vi "SaveMean_Example.vi"() -> ()   [LabVIEW 2019]
doc: "This example shows how to record an image sequence, get the mean of that sequence and save it to file afterwards.\nIt is a good starting point for writing own applications.\nBut it will not be fail save, i.e. doesnt react on errors, just handles them forward to the end\n\nUsage:\nSelect your required image count you want to average over before you start the program.\nOnce started, the camera class will be initialized and images will be recorded automatically.\nTWhen acquisition has finished the mean image is read and shown.\nNow you can crop the image using the ROI parameters and select a file path.\nBy clicking save, the mean image is saved with the selected file format using the current roi setting\nThis also finishes the program and will force an exit of the camera class"
uses:
  camera/Camera.lvclass
  pco.recorder/Recorder.lvlib
  <vilib>/picture/picture.llb/Draw 8-Bit Pixmap.vi
  <vilib>/picture/picture.llb/Draw True-Color Pixmap.vi
panel:
  out "colormap(U8)":u32[](array[numeric])
  out "Image(U16)":u16[][](graph)
  in  "Zoom [%]":i32(slide)=26 min=10 max=200 step=5 scale=10.0..200.0
  out "Image":picture
  out "rawImage":u16[][](array[numeric])
  in  "data_format":T1(ring)=enum."Mono16"
  in  "Image Index":u32 max=99
  in  "saveImages":bool
  in  "SavePath":path
  out "Recorded Images":u32
  in  "Quit":bool
  in  "cropY1":u64=2 min=2 max=2048 step=1
  in  "cropX1":u64=2 min=2 max=2048 step=1
  in  "cropY0":u64=1 min=1 max=2047 step=1
  in  "cropX0":u64=1 min=1 max=2047 step=1
  out "Image Height":u16
  out "Image Width":u16
  in  "dwImgCount":u32=10 caption="Required Number of Images" max=4023
  out "Error":errorcluster {"code" format="%x"}
  # "This example shows how to record an image sequence, get the mean of that sequence and save it to file afterwards.\nIt is a good starting point for writing own applications.\nBut it will not be fail save, i.e. doesnt react on errors, just handles them forward to the end\n\nUsage:\nSelect your required image count you want to average over before you start the program.\nOnce started, the camera class will be initialized and images will be recorded automatically.\nTWhen acquisition has finished the mean image is read and shown.\nNow you can crop the image using the crop parameters and select a file path.\nBy clicking save, the mean image is saved with the selected file format using the current roi setting\nThis also finishes the program and will force an exit of the camera class"
  # "pco.labview"
  # "Camera Setup"
  # "Recording Control"
  # "Parameters for image readout"
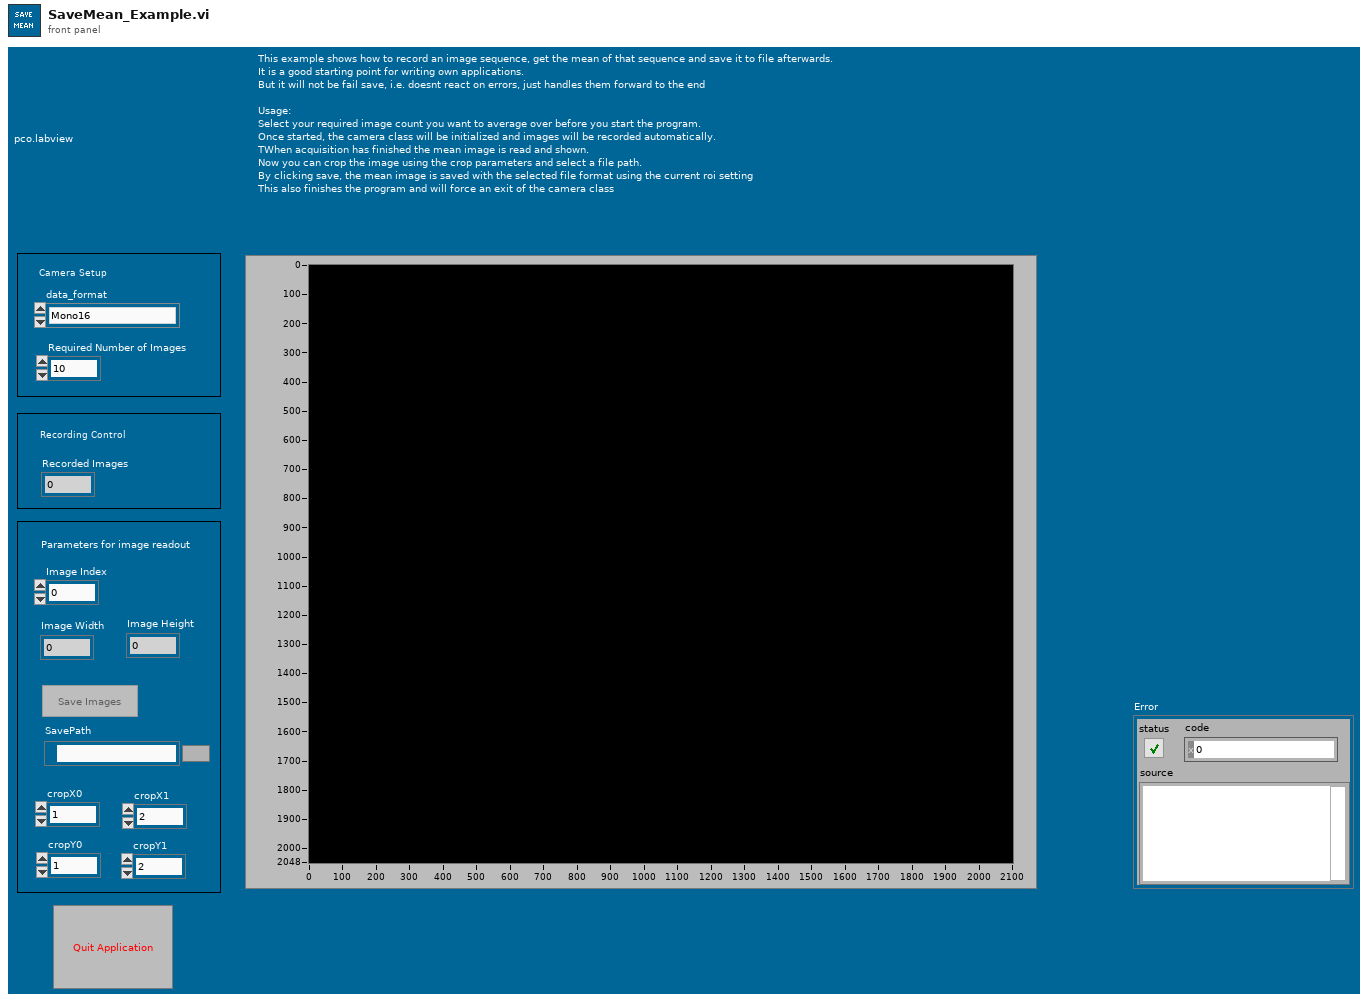
[diagram p1: front panel]
types:
  T1 = enum16{"Undefined", "Mono8", "Mono16", "BGRA8", "RGBA8", "BGRA16", "RGBA16", "CompressedMono8"}
  T2 = enum8{"Enabled", "Disabled", "Disabled and Grayed Out"}
  T3 = enum16{"sequence", "sequence non blocking", "ring buffer", "fifo", "tif", "multitif", "pcoraw", "b16", "dicom", "multidicom", "camram_ring", "camram_segment"}
  T4 = cluster{"wVersion":u16, "dwIMAGE_COUNTER":u32, "dwIMAGE_TIME_US":u32, "lvTimestamp":timestamp, "bIMAGE_TIME_STATUS":u8, "wEXPOSURE_TIME_BASE":u16, "dwEXPOSURE_TIME":u32, "dwFRAMERATE_MILLIHZ":u32, "sSENSOR_TEMPERATURE":i16, "wIMAGE_SIZE_X":u16, "wIMAGE_SIZE_Y":u16, "bBINNING_X":u8, "bBINNING_Y":u8, "dwSENSOR_READOUT_FREQUENCY":u32, "wSENSOR_CONV_FACTOR":u16, "dwCAMERA_SERIAL_NO":u32, "wCAMERA_TYPE":u16, "bBIT_RESOLUTION":u8, "bSYNC_STATUS":u8, "wDARK_OFFSET":u16, "bTRIGGER_MODE":u8, "bDOUBLE_IMAGE_MODE":u8, "bCAMERA_SYNC_MODE":u8, "bIMAGE_TYPE":u8, "wCOLOR_PATTERN":u16, "wCAMERA_SUBTYPE":u16, "dwEVENT_NUMBER":u32, "wIMAGE_SIZE_X_Offset":u16, "wIMAGE_SIZE_Y_Offset":u16, "bREADOUT_MODE":u8}
  T5 = typedef "Camera.lvclass/binning.ctl" = cluster{"vert":u16, "horz":u16, "mode":u16}
  T6 = cluster{"exposure_time_s":dbl, "delay_time_s":dbl, "roi":cluster{"x0":u64, "y0":u64, "x1":u64, "y1":u64}, "timestamp_mode":u16, "pixelrate":u32, "conversion_factor":sgl, "trigger_mode":u16, "acquire_mode":u16, "acquire_sequence_number":u32, "metadata_mode":u16, "noisefilter_mode":u16, "pixel_format":u32, "binning":T5, "auto_exposure":cluster{"region":u16, "min_exposure_s":dbl, "max_exposure_s":dbl}}
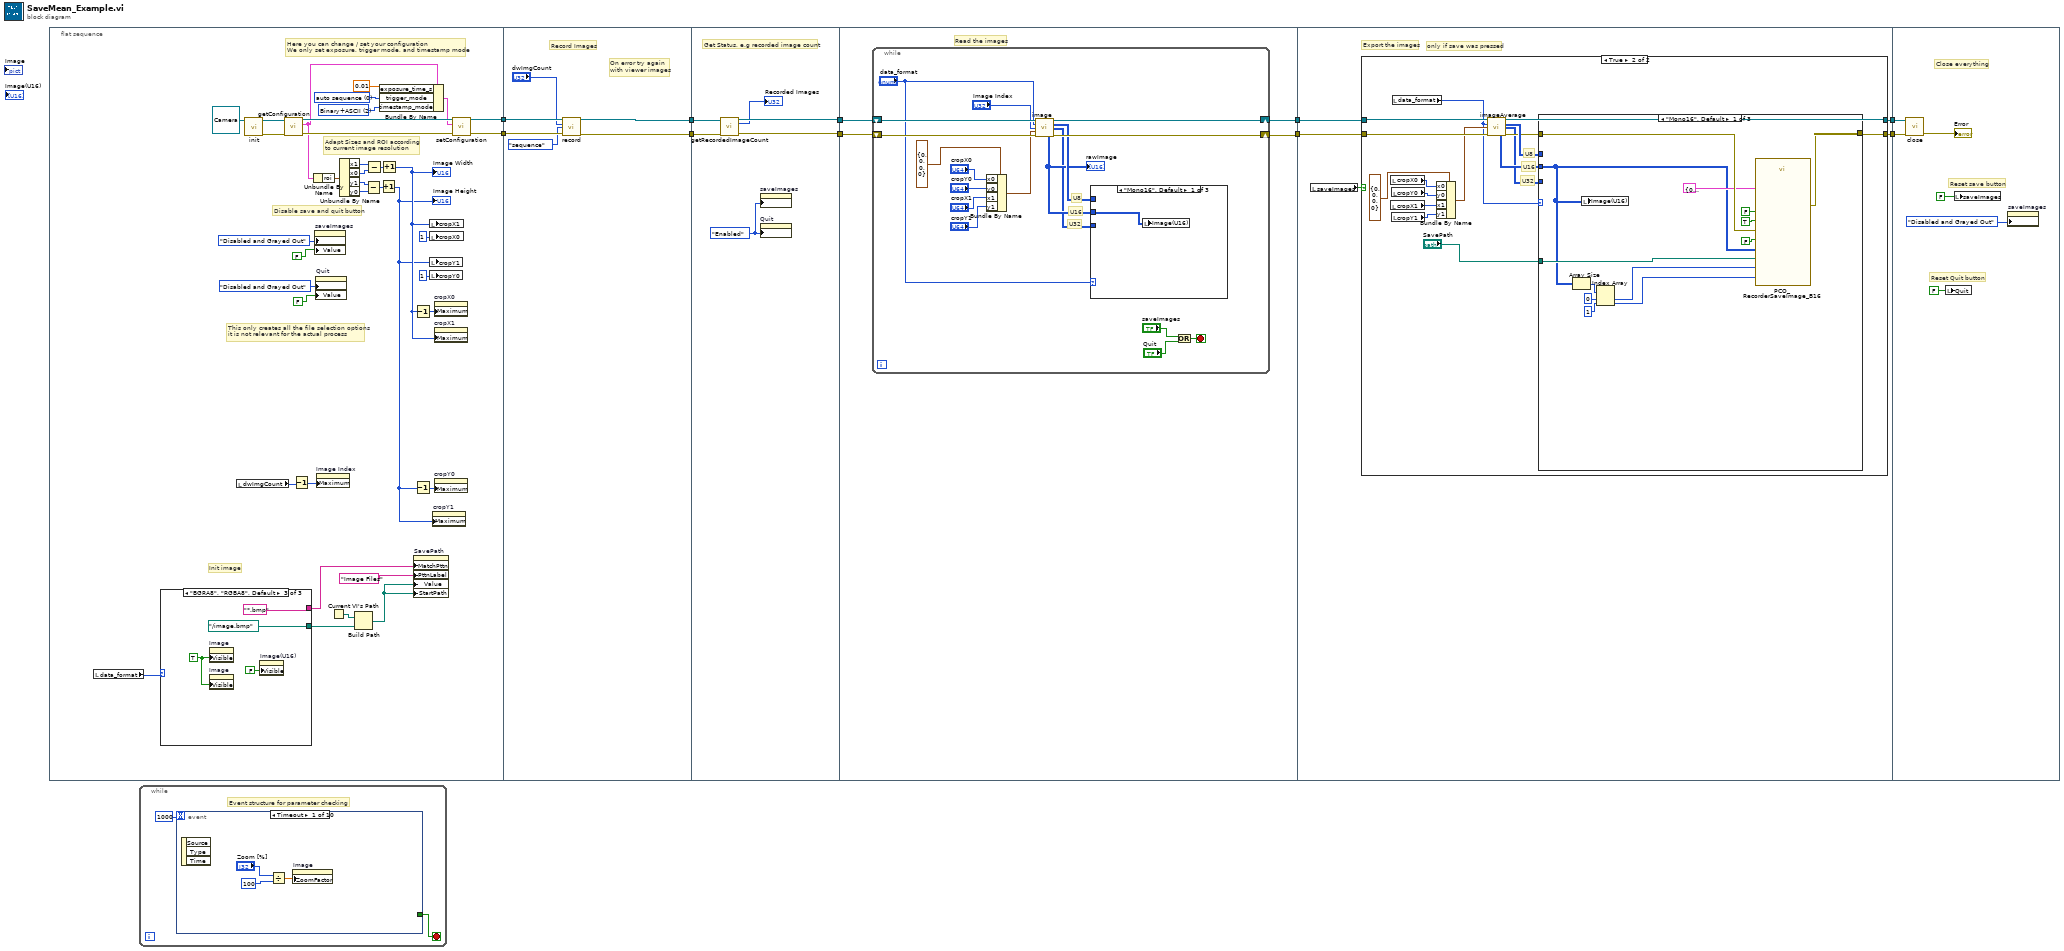
[diagram p0: block diagram]
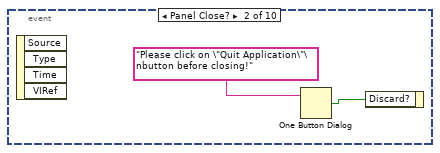
[diagram p2: hidden frame]
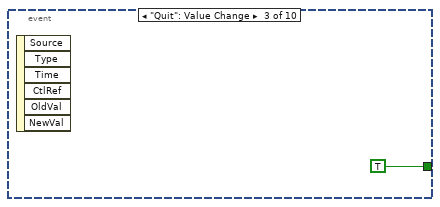
[diagram p3: hidden frame]
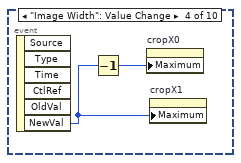
[diagram p4: hidden frame]
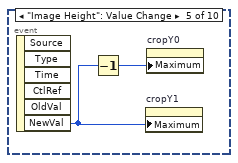
[diagram p5: hidden frame]
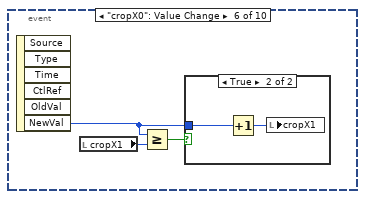
[diagram p6: hidden frame]
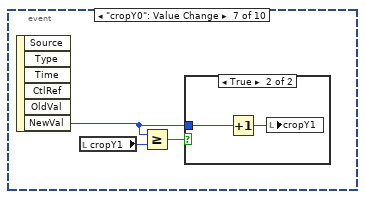
[diagram p8: hidden frame]
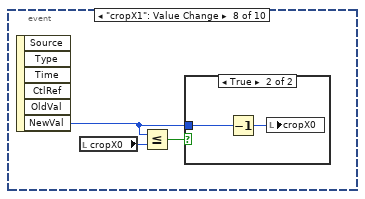
[diagram p10: hidden frame]
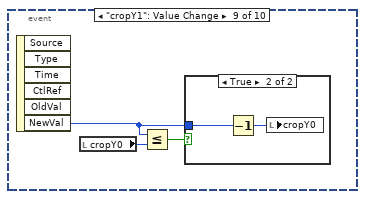
[diagram p12: hidden frame]
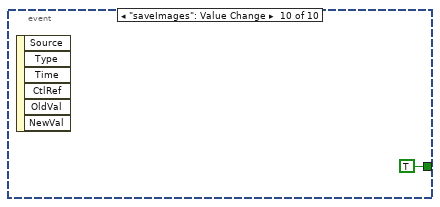
[diagram p14: hidden frame]
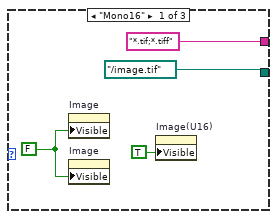
[diagram p15: hidden frame]
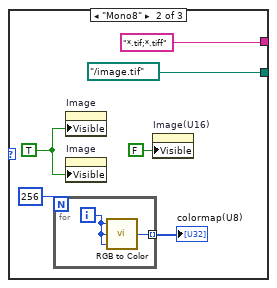
[diagram p16: hidden frame]
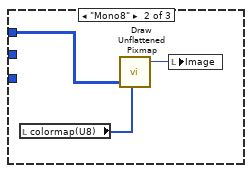
[diagram p17: hidden frame]
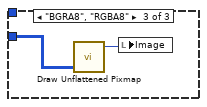
[diagram p18: hidden frame]
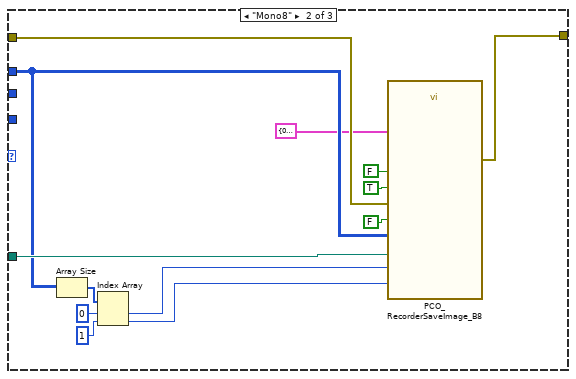
[diagram p20: hidden frame]
diagram:
  n1 = flat-sequence {
    tunnel: [w38] -> w10
    tunnel: [w37] -> w9
    tunnel: w10 -> [w69]
    tunnel: w9 -> [w68]
    tunnel: [w66] -> w8
    tunnel: [w65] -> w7
    tunnel: w8 -> [w75]
    tunnel: w7 -> [w74]
    tunnel: [w73] -> w6
    tunnel: [w72] -> w5
    tunnel: w6 -> [w78]
    tunnel: w5 -> [w79]
    tunnel: [w77] -> w4
    tunnel: [w76] -> w2
    tunnel: w4 -> [w107]
    tunnel: [w106] -> w3
    tunnel: w2 -> [w105]
    tunnel: [w104] -> w1
    tunnel: w3 -> [w180]
    tunnel: w1 -> [w179]
    frame #0 {
      w22 = u16 2 items=["OFF", "Binary", "Binary+ASCII", "ASCII"] ("TimestampMode")
      w44 = u16 0 items=["auto sequence"=0, "software trigger"=1, "external exposure start & software trigger"=2, "external exposure control"=3, "external synchronized"=4, "fast external exposure control"=5, "external CDS control"=6, "slow external exposure control"=7, "external synchronized HDSDI"=258] ("TriggerMode")
      # "Here you can change / set your configuration\nWe only set exposure, trigger mode, and timestamp mode"
      # "Init image"
      # "This only creates all the file selection options\nit is not relevant for the actual process"
      # "Adapt Sizes and ROI according\nto current image resolution"
      # "Disable save and quit button"
      n2 = local read "data_format"() -> (w14:T1)
      n3 = case shown="\"BGRA8\", \"RGBA8\", Default" w14 {
        tunnel: [path "../image.tif" ("SavePath") path "../image.tif" ("SavePath") path "../image.bmp" ("SavePath")] -> w13
        tunnel: ["*.tif;*.tiff" ("pattern (all files)") "*.tif;*.tiff" ("pattern (all files)") "*.bmp" ("pattern (all files)")] -> w12
        frame "Mono16" {
          w50 = FALSE ("Visible")
          n4 = property on="Image" class="Pict"("Visible"=w50) -> ()  [unwired: 2 in, 2 out]
          n5 = property on="Image" class="Pict"("Visible"=w50) -> ()  [unwired: 2 in, 2 out]
          n6 = property on="Image(U16)" class="IntGraph (strict)"("Visible"=TRUE) -> ()  [unwired: 2 in, 2 out]
        }
        frame "Mono8" {
          w56 = TRUE ("Visible")
          n7 = for {
            N: 256 -> [_]
            tunnel: [w58] -> w55 mode=indexing
            i -> [w59]
            n8 = call <vilib>:"RGB to Color.vi"("B"=w59, "G"=w59, "R"=w59) -> ("Color"=w58:u32)
          }
          "colormap(U8)" <- w55
          n9 = property on="Image" class="Pict"("Visible"=w56) -> ()  [unwired: 2 in, 2 out]
          n10 = property on="Image" class="Pict"("Visible"=w56) -> ()  [unwired: 2 in, 2 out]
          n11 = property on="Image(U16)" class="IntGraph (strict)"("Visible"=FALSE) -> ()  [unwired: 2 in, 2 out]
        }
        frame "BGRA8", "RGBA8", Default {
          w63 = TRUE ("Visible")
          n12 = property on="Image" class="Pict"("Visible"=w63) -> ()  [unwired: 2 in, 2 out]
          n13 = property on="Image" class="Pict"("Visible"=w63) -> ()  [unwired: 2 in, 2 out]
          n14 = property on="Image(U16)" class="IntGraph (strict)"("Visible"=FALSE) -> ()  [unwired: 2 in, 2 out]
        }
      }
      n15 = local read "dwImgCount"() -> (w15:u32)
      n16 = call-dynamic "init.vi"("Camera in"=refnum<class "Camera.lvclass"> refnum ("PCOCamera in")) -> ("Camera out"=w46:refnum<class "Camera.lvclass">, "error out"=w45:errorcluster)  [unwired: 8 in]
      n17 = call-dynamic "getConfiguration.vi"("error in (no error)"=w45, "Camera in"=w46) -> ("error out"=w42:errorcluster, "configuration"=w32:T6, "Camera out"=w43:refnum<class "Camera.lvclass">)  [unwired: 7 in]
      n18 = Decrement(x=w15) -> (x-1=w16:u32)
      n19 = Unbundle By Name(w32) -> ("roi"=w31:cluster{"x0":u64, "y0":u64, "x1":u64, "y1":u64})
      n20 = property on="saveImages" class="Bool (strict)"("DisabledEnum"=T2."Disabled and Grayed Out" ("Disabled"), "Value"=FALSE ("Stop")) -> ()  [unwired: 2 in, 2 out]
      n21 = property on="Quit" class="Bool (strict)"("DisabledEnum"=T2."Disabled and Grayed Out" ("Disabled"), "Value"=FALSE ("Stop")) -> ()  [unwired: 2 in, 2 out]
      n22 = property on="Image Index" class="DigNum (strict)"("Maximum"=w16) -> ()  [unwired: 2 in, 2 out]
      n23 = Current VI's Path() -> (path=w19:path)
      n24 = Unbundle By Name(w31) -> ("x1"=w29:u64, "x0"=w30:u64, "y1"=w27:u64, "y0"=w28:u64)
      n25 = Build Path(base path=w19, name or relative path=w13) -> (appended path=w17:path)
      n26 = Subtract(x=w27, y=w28) -> (x-y=w25:u64)
      n27 = Subtract(x=w29, y=w30) -> (x-y=w26:u64)
      n28 = Bundle By Name(cluster=w32, "exposure_time_s"=0.01, "trigger_mode"=w44, "timestamp_mode"=w22) -> (w41:T6)
      n29 = Increment(x=w25) -> (x+1=w23:u64)
      "Image Height" <- w23
      n30 = Increment(x=w26) -> (x+1=w24:u64)
      "Image Width" <- w24
      n31 = property on="SavePath" class="Path"("MatchPttn"=w12, "PttnLabel"="Image Files" ("pattern label"), "Value"=w17, "StartPath"=w17) -> ()  [unwired: 2 in, 2 out]
      n32 = Decrement(x=w24) -> (x-1=w34:u64)
      n33 = Decrement(x=w23) -> (x-1=w33:u64)
      n34 = local write "cropX1"(w24) -> ()
      n35 = local write "cropX0"(u16 1 ("roiY0")) -> ()
      n36 = local write "cropY1"(w23) -> ()
      n37 = local write "cropY0"(u16 1 ("roiY0")) -> ()
      n38 = property on="cropY1" class="DigNum (strict)"("Maximum"=w23) -> ()  [unwired: 2 in, 2 out]
      n39 = property on="cropX0" class="DigNum (strict)"("Maximum"=w34) -> ()  [unwired: 2 in, 2 out]
      n40 = property on="cropX1" class="DigNum (strict)"("Maximum"=w24) -> ()  [unwired: 2 in, 2 out]
      n41 = property on="cropY0" class="DigNum (strict)"("Maximum"=w33) -> ()  [unwired: 2 in, 2 out]
      n42 = call-dynamic "setConfiguration.vi"("error in (no error)"=w42, "configuration"=w41, "Camera in"=w43) -> ("error out"=w37:errorcluster, "Camera out"=w38:refnum<class "Camera.lvclass">)  [unwired: 7 in]
    }
    frame #1 {
      # "On error try again \nwith viewer images"
      # "Record Images"
      n43 = call-dynamic "record.vi"("Camera in"=w69, "num_images"="dwImgCount", "record_mode"=T3."sequence", "error in (no error)"=w68) -> ("Camera out"=w66:refnum<class "Camera.lvclass">, "error out"=w65:errorcluster)  [unwired: 10 in]
    }
    frame #2 {
      w70 = T2."Enabled" ("Disabled")
      # "Get Status, e.g recorded image count"
      n44 = call-dynamic "getRecordedImageCount.vi"("Camera in"=w75, "error in (no error)"=w74) -> ("Camera out"=w73:refnum<class "Camera.lvclass">, "recorded_image_count"=→"Recorded Images":u32, "error out"=w72:errorcluster)  [unwired: 11 in]
      n45 = property on="saveImages" class="Bool (strict)"("DisabledEnum"=w70) -> ()  [unwired: 2 in, 2 out]
      n46 = property on="Quit" class="Bool (strict)"("DisabledEnum"=w70) -> ()  [unwired: 2 in, 2 out]
    }
    frame #3 {
      # "Read the images"
      n47 = while {
        shift-right: [w95] -> w77
        shift-left: w78 -> [w97]
        shift-right: [w90] -> w76
        shift-left: w79 -> [w96]
        stop <- w88 stop-if-true
        # "U32"
        # "U16"
        # "U8"
        n48 = Bundle By Name(cluster=cluster{"x0":u64, "y0":u64, "x1":u64, "y1":u64} {"x0"=0, "y0"=0, "x1"=0, "y1"=0} ("roi"), "x0"="cropX0", "y0"="cropY0", "x1"="cropX1", "y1"="cropY1") -> (w86:cluster{"x0":u64, "y0":u64, "x1":u64, "y1":u64})
        n49 = call-dynamic "image.vi"("Camera in"=w97, "data_format"="data_format", "image_index"="Image Index", "crop"=w86, "error in (no error)"=w96) -> ("Camera out"=w95:refnum<class "Camera.lvclass">, "image (U8)"=w83:u8[][], "image (U32)"=w81:u32[][], "raw_image (U16)"=w82:u16[][], "error out"=w90:errorcluster)  [unwired: 2 in, 4 out]
        "rawImage" <- w82
        n50 = case shown="\"Mono16\", Default" "data_format" {
          tunnel: w81 -> [_ _ w103]
          tunnel: w83 -> [_ w101 _]
          tunnel: w82 -> [w98 _ _]
          frame "Mono16", Default {
            n51 = local write "Image(U16)"(w98) -> ()
          }
          frame "Mono8" {
            n52 = local read "colormap(U8)"() -> (w100:u32[])
            n53 = call-poly <vilib>:"Draw Unflattened Pixmap.vi"("data"=w101, "color table"=w100) -> ("new picture"=w99:picture)  [unwired: 7 in]
            n54 = local write "Image"(w99) -> ()
          }
          frame "BGRA8", "RGBA8" {
            n55 = call-poly <vilib>:"Draw Unflattened Pixmap.vi"("data (RGB format)"=w103) -> ("new picture"=w102:picture)  [unwired: 8 in]
            n56 = local write "Image"(w102) -> ()
          }
        }
        n57 = Or(x="saveImages", y="Quit") -> (x .or. y?=w88:bool)
      }
    }
    frame #4 {
      # "only if save was pressed"
      # "Export the images"
      n58 = local read "saveImages"() -> (w108:bool)
      n59 = case shown="True" w108 {
        tunnel: w107 -> [w110 w125]
        tunnel: [w110 w116] -> w106
        tunnel: w105 -> [w109 w126]
        tunnel: [w109 w112] -> w104
        frame False {
        }
        frame True {
          # "U32"
          # "U16"
          # "U8"
          n60 = local read "cropX0"() -> (w123:u64)
          n61 = local read "cropX1"() -> (w121:u64)
          n62 = local read "cropY0"() -> (w122:u64)
          n63 = local read "cropY1"() -> (w120:u64)
          n64 = local read "data_format"() -> (w115:T1)
          n65 = Bundle By Name(cluster=cluster{"x0":u64, "y0":u64, "x1":u64, "y1":u64} {"x0"=0, "y0"=0, "x1"=0, "y1"=0} ("roi"), "x0"=w123, "y0"=w122, "x1"=w121, "y1"=w120) -> (w119:cluster{"x0":u64, "y0":u64, "x1":u64, "y1":u64})
          n66 = call-dynamic "imageAverage.vi"("Camera in"=w125, "data_format"=w115, "crop"=w119, "error in (no error)"=w126) -> ("Camera out"=w116:refnum<class "Camera.lvclass">, "image (U8)"=w118:u8[][], "image (U32)"=w111:u32[][], "raw_image (U16)"=w117:u16[][], "error out"=w113:errorcluster)  [unwired: 5 in, 2 out]
          n67 = case shown="\"Mono16\", Default" w115 {
            tunnel: w111 -> [_ _ w156]
            tunnel: w118 -> [_ w143 _]
            tunnel: w117 -> [w127 _ _]
            tunnel: "SavePath" -> [w134 w149 w174]
            tunnel: w113 -> [w136 w148 w172]
            tunnel: [w135 w147 w171] -> w112
            frame "Mono16", Default {
              n68 = Array Size(array=w127) -> (size(s)=w133:i32[])
              n69 = local write "Image(U16)"(w127) -> ()
              n70 = Index Array(array=w133, index #1=0 ("index"), index #2=1 ("index")) -> (element #1=w130:i32, element #2=w129:i32)
              n71 = call "PCO_RecorderSaveImage_B16.vi"("pImgBuf"=w127, "wWidth"=w129, "wHeight"=w130, "szFilePath"=w134, "error in (no error)"=w136, "isColor"=FALSE, "bIsBitmap"=FALSE, "PCO_METADATA_STRUCT"=T4 {"wVersion"=0, "dwIMAGE_COUNTER"=0, "dwIMAGE_TIME_US"=0, "lvTimestamp"=timestamp(0 s since 1904-01-01), "bIMAGE_TIME_STATUS"=0, "wEXPOSURE_TIME_BASE"=0, "dwEXPOSURE_TIME"=0, "dwFRAMERATE_MILLIHZ"=0, "sSENSOR_TEMPERATURE"=0, "wIMAGE_SIZE_X"=0, "wIMAGE_SIZE_Y"=0, "bBINNING_X"=0, "bBINNING_Y"=0, "dwSENSOR_READOUT_FREQUENCY"=0, "wSENSOR_CONV_FACTOR"=0, "dwCAMERA_SERIAL_NO"=0, "wCAMERA_TYPE"=0, "bBIT_RESOLUTION"=0, "bSYNC_STATUS"=0, "wDARK_OFFSET"=0, "bTRIGGER_MODE"=0, "bDOUBLE_IMAGE_MODE"=0, "bCAMERA_SYNC_MODE"=0, "bIMAGE_TYPE"=0, "wCOLOR_PATTERN"=0, "wCAMERA_SUBTYPE"=0, "dwEVENT_NUMBER"=0, "wIMAGE_SIZE_X_Offset"=0, "wIMAGE_SIZE_Y_Offset"=0, "bREADOUT_MODE"=0}, "bOverwrite"=TRUE) -> ("error out"=w135:errorcluster)  [unwired: 9 in, 1 out]
            }
            frame "Mono8" {
              n72 = Array Size(array=w143) -> (size(s)=w146:i32[])
              n73 = Index Array(array=w146, index #1=0 ("index"), index #2=1 ("index")) -> (element #1=w142:i32, element #2=w141:i32)
              n74 = call "PCO_RecorderSaveImage_B8.vi"("pImgBuf"=w143, "wWidth"=w141, "wHeight"=w142, "szFilePath"=w149, "error in (no error)"=w148, "isColor"=FALSE, "bIsBitmap"=FALSE, "PCO_METADATA_STRUCT"=T4 {"wVersion"=0, "dwIMAGE_COUNTER"=0, "dwIMAGE_TIME_US"=0, "lvTimestamp"=timestamp(0 s since 1904-01-01), "bIMAGE_TIME_STATUS"=0, "wEXPOSURE_TIME_BASE"=0, "dwEXPOSURE_TIME"=0, "dwFRAMERATE_MILLIHZ"=0, "sSENSOR_TEMPERATURE"=0, "wIMAGE_SIZE_X"=0, "wIMAGE_SIZE_Y"=0, "bBINNING_X"=0, "bBINNING_Y"=0, "dwSENSOR_READOUT_FREQUENCY"=0, "wSENSOR_CONV_FACTOR"=0, "dwCAMERA_SERIAL_NO"=0, "wCAMERA_TYPE"=0, "bBIT_RESOLUTION"=0, "bSYNC_STATUS"=0, "wDARK_OFFSET"=0, "bTRIGGER_MODE"=0, "bDOUBLE_IMAGE_MODE"=0, "bCAMERA_SYNC_MODE"=0, "bIMAGE_TYPE"=0, "wCOLOR_PATTERN"=0, "wCAMERA_SUBTYPE"=0, "dwEVENT_NUMBER"=0, "wIMAGE_SIZE_X_Offset"=0, "wIMAGE_SIZE_Y_Offset"=0, "bREADOUT_MODE"=0}, "bOverwrite"=TRUE) -> ("error out"=w147:errorcluster)  [unwired: 9 in, 1 out]
            }
            frame "BGRA8", "RGBA8" {
              # "We need A channel at the end"
              n75 = Array Size(array=w156) -> (size(s)=w159:i32[])
              n76 = Index Array(array=w159, index #1=0 ("index"), index #2=1 ("index")) -> (element #1=w155:i32, element #2=w154:i32)
              n77 = Rotate(1:w156, 2:i16 8 ("y")) -> (0:w160:u32[][])
              n78 = Multiply(x=w155, y=w154) -> (x*y=w165:i32)
              n79 = Reshape Array(w160, w165) -> (w166:u32[])
              n80 = Multiply(x=w154, y=u64 4) -> (x*y=w167:u64)
              n81 = Type Cast(type=u8[] [] ("image_list (U32)"), x=w166) -> (*(type *) &x=w168:u8[])
              n82 = Reshape Array(w168, w155, w167) -> (w162:u8[][])
              n83 = call "PCO_RecorderSaveImage_B8.vi"("pImgBuf"=w162, "wWidth"=w154, "wHeight"=w155, "szFilePath"=w174, "error in (no error)"=w172, "isColor"=TRUE, "bIsBitmap"=FALSE, "PCO_METADATA_STRUCT"=T4 {"wVersion"=0, "dwIMAGE_COUNTER"=0, "dwIMAGE_TIME_US"=0, "lvTimestamp"=timestamp(0 s since 1904-01-01), "bIMAGE_TIME_STATUS"=0, "wEXPOSURE_TIME_BASE"=0, "dwEXPOSURE_TIME"=0, "dwFRAMERATE_MILLIHZ"=0, "sSENSOR_TEMPERATURE"=0, "wIMAGE_SIZE_X"=0, "wIMAGE_SIZE_Y"=0, "bBINNING_X"=0, "bBINNING_Y"=0, "dwSENSOR_READOUT_FREQUENCY"=0, "wSENSOR_CONV_FACTOR"=0, "dwCAMERA_SERIAL_NO"=0, "wCAMERA_TYPE"=0, "bBIT_RESOLUTION"=0, "bSYNC_STATUS"=0, "wDARK_OFFSET"=0, "bTRIGGER_MODE"=0, "bDOUBLE_IMAGE_MODE"=0, "bCAMERA_SYNC_MODE"=0, "bIMAGE_TYPE"=0, "wCOLOR_PATTERN"=0, "wCAMERA_SUBTYPE"=0, "dwEVENT_NUMBER"=0, "wIMAGE_SIZE_X_Offset"=0, "wIMAGE_SIZE_Y_Offset"=0, "bREADOUT_MODE"=0}, "bOverwrite"=TRUE) -> ("error out"=w171:errorcluster)  [unwired: 9 in, 1 out]
            }
          }
        }
      }
    }
    frame #5 {
      # "Reset Quit button"
      # "Close everything"
      # "Reset save button"
      n84 = call-dynamic "close.vi"("error in (no error)"=w179, "Camera in"=w180) -> ("error out"=→"Error":errorcluster)  [unwired: 9 in]
      n85 = local write "Quit"(FALSE ("Stop")) -> ()
      n86 = local write "saveImages"(FALSE ("Stop")) -> ()
      n87 = property on="saveImages" class="Bool (strict)"("DisabledEnum"=T2."Disabled and Grayed Out" ("Disabled")) -> ()  [unwired: 2 in, 2 out]
    }
  }
  n88 = while {
    stop <- w181 stop-if-true
    # "Event structure for parameter checking"
    n89 = event shown="[0] Timeout" {
      selector: _ -> [_ _ _ _ _ _ _ _ _ _]
      dyn-events: _ -> [_ _ _ _ _ _ _ _ _ _]
      timeout: 1000 -> [_ _ _ _ _ _ _ _ _ _]
      tunnel: [_ _ TRUE _ _ _ _ _ _ TRUE] -> w181
      event Timeout {
        n90 = event-data() -> ()  [unwired: 1 in, 3 out]
        n91 = Divide(x="Zoom [%]", y=100 ("Zoom [%]")) -> (x/y=w185:dbl)
        n92 = property on="Image" class="Pict"("ZoomFactor"=w185) -> ()  [unwired: 2 in, 2 out]
      }
      event Panel Close? {
        n93 = event-data() -> ()  [unwired: 1 in, 4 out]
        n94 = One Button Dialog(message="Please click on \"Quit Application\"\nbutton before closing!") -> (true=w186:bool)  [unwired: 1 in]
        n95 = event-data("Discard?"=w186) -> ()  [unwired: 1 in, 1 out]
      }
      event "Quit": Value Change {
        n96 = event-data() -> ()  [unwired: 1 in, 6 out]
      }
      event "Image Width": Value Change {
        n97 = event-data() -> ("NewVal"=w189:u16)  [unwired: 1 in, 5 out]
        n98 = Decrement(x=w189) -> (x-1=w190:u16)
        n99 = property on="cropX0" class="DigNum (strict)"("Maximum"=w190) -> ()  [unwired: 2 in, 2 out]
        n100 = property on="cropX1" class="DigNum (strict)"("Maximum"=w189) -> ()  [unwired: 2 in, 2 out]
      }
      event "Image Height": Value Change {
        n101 = event-data() -> ("NewVal"=w191:u16)  [unwired: 1 in, 5 out]
        n102 = Decrement(x=w191) -> (x-1=w192:u16)
        n103 = property on="cropY1" class="DigNum (strict)"("Maximum"=w191) -> ()  [unwired: 2 in, 2 out]
        n104 = property on="cropY0" class="DigNum (strict)"("Maximum"=w192) -> ()  [unwired: 2 in, 2 out]
      }
      event "cropX0": Value Change {
        n105 = event-data() -> ("NewVal"=w193:u64)  [unwired: 1 in, 5 out]
        n106 = local read "cropX1"() -> (w195:u64)
        n107 = Greater Or Equal?(x=w193, y=w195) -> (x >= y?=w194:bool)
        n108 = case shown="True" w194 {
          tunnel: w193 -> [_ w197]
          frame False {
          }
          frame True {
            n109 = Increment(x=w197) -> (x+1=w196:u64)
            n110 = local write "cropX1"(w196) -> ()
          }
        }
      }
      event "cropY0": Value Change {
        n111 = event-data() -> ("NewVal"=w198:u64)  [unwired: 1 in, 5 out]
        n112 = local read "cropY1"() -> (w200:u64)
        n113 = Greater Or Equal?(x=w198, y=w200) -> (x >= y?=w199:bool)
        n114 = case shown="True" w199 {
          tunnel: w198 -> [_ w202]
          frame False {
          }
          frame True {
            n115 = Increment(x=w202) -> (x+1=w201:u64)
            n116 = local write "cropY1"(w201) -> ()
          }
        }
      }
      event "cropX1": Value Change {
        n117 = event-data() -> ("NewVal"=w203:u64)  [unwired: 1 in, 5 out]
        n118 = local read "cropX0"() -> (w205:u64)
        n119 = Less Or Equal?(x=w203, y=w205) -> (x <= y?=w204:bool)
        n120 = case shown="True" w204 {
          tunnel: w203 -> [_ w207]
          frame False {
          }
          frame True {
            n121 = Decrement(x=w207) -> (x-1=w206:u64)
            n122 = local write "cropX0"(w206) -> ()
          }
        }
      }
      event "cropY1": Value Change {
        n123 = event-data() -> ("NewVal"=w208:u64)  [unwired: 1 in, 5 out]
        n124 = local read "cropY0"() -> (w210:u64)
        n125 = Less Or Equal?(x=w208, y=w210) -> (x <= y?=w209:bool)
        n126 = case shown="True" w209 {
          tunnel: w208 -> [_ w212]
          frame False {
          }
          frame True {
            n127 = Decrement(x=w212) -> (x-1=w211:u64)
            n128 = local write "cropY0"(w211) -> ()
          }
        }
      }
      event "saveImages": Value Change {
        n129 = event-data() -> ()  [unwired: 1 in, 6 out]
      }
    }
  }
